vi "EOL Truncate Number.vi"(9 "Desired Decimal Points":u8=2, 10 "truncate instead of round":bool, 11 "Numeric Input":sgl format="%#_11g") -> (3 "Numeric Output":sgl)   [LabVIEW 2018]
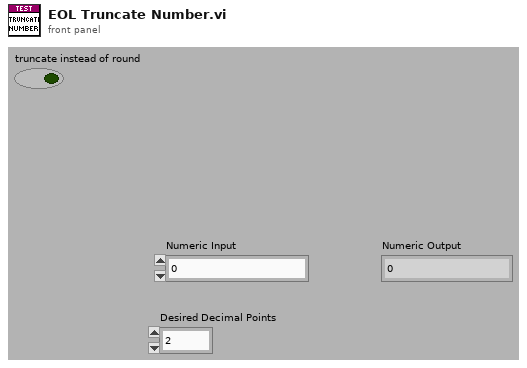
[diagram p1: front panel]
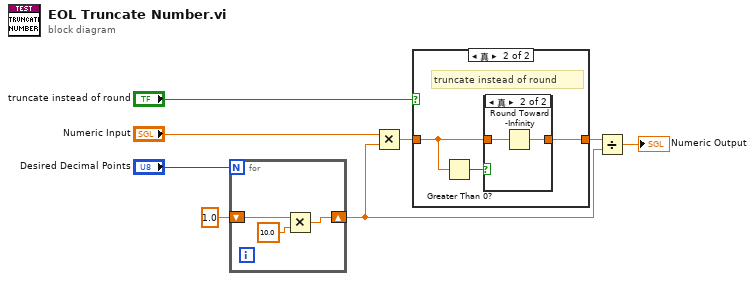
[diagram p0: block diagram]
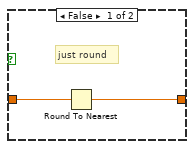
[diagram p2: hidden frame]
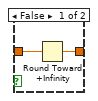
[diagram p3: hidden frame]
diagram:
  n1 = for {
    N: "Desired Decimal Points" -> [_]
    shift-right: [w11] -> w3
    shift-left: sgl 1.0 ("y") -> [w9]
    n2 = Multiply(x=w9, y=sgl 10.0) -> (x*y=w11:sgl)
  }
  n3 = Multiply(x="Numeric Input", y=w3) -> (x*y=w5:sgl)
  n4 = case shown="真" "truncate instead of round" {
    tunnel: w5 -> [w13 w15]
    tunnel: [w12 w14] -> w4
    frame False {
      # "just round"
      n5 = Round To Nearest(number=w13) -> (nearest integer value=w12:sgl)
    }
    frame True {
      # "truncate instead of round"
      n6 = Greater Than 0?(x=w15) -> (x > 0?=w16:bool)
      n7 = case shown="真" w16 {
        tunnel: w15 -> [w18 w20]
        tunnel: [w17 w19] -> w14
        frame False {
          n8 = Round Toward +Infinity(x=w18) -> (ceil(x): smallest int >= x=w17:sgl)
        }
        frame True {
          n9 = Round Toward -Infinity(1:w20) -> (0:w19:sgl)
        }
      }
    }
  }
  n10 = Divide(x=w4, y=w3) -> (x/y=→"Numeric Output":sgl)
